vi "startup.vi"(8 "error in (no error)":errorcluster, 11 "ActionEditor in":refnum<class "ActionEditor.lvclass">) -> (0 "error out":errorcluster, 3 "ActionEditor out":refnum<class "ActionEditor.lvclass">)   [LabVIEW 2011, in "Views.lvlib" / "ScriptEditor.lvlib" / "ActionEditor.lvclass"]
uses:
  ActionEditor.lvclass
  ActionEditor.lvclass/ActionEditor.ctl
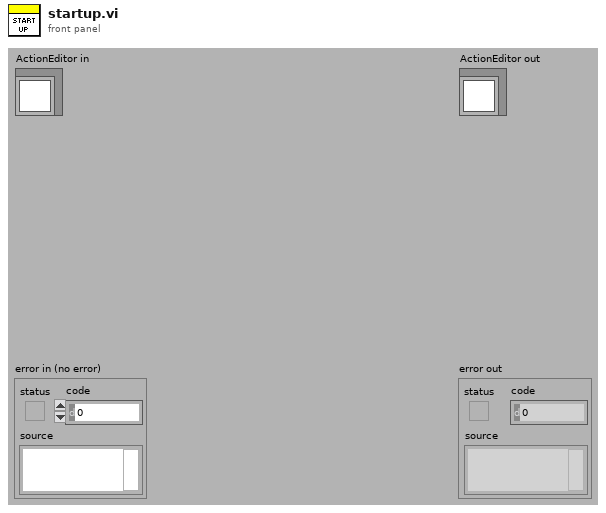
[diagram p1: front panel]
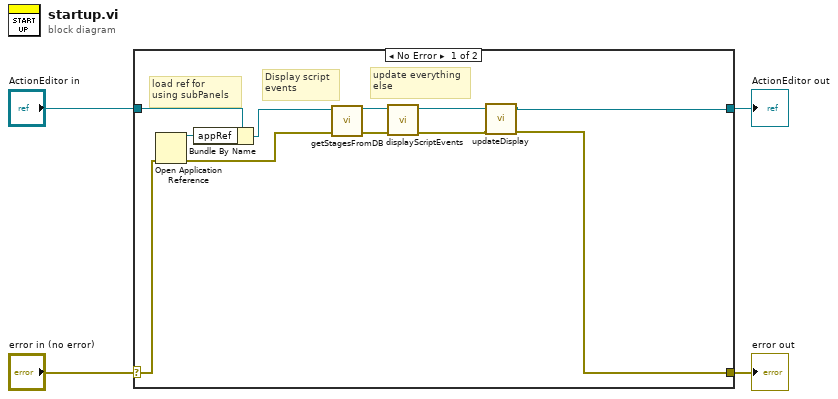
[diagram p0: block diagram]
diagram:
  n1 = case shown="No Error" "error in (no error)" {
    selector: "error in (no error)" -> [w12 w16]
    tunnel: [w7 w16] -> w3
    tunnel: [w8 w15] -> w1
    tunnel: "ActionEditor in" -> [w14 w15]
    frame No Error {
      # "update everything\nelse"
      # "Display script \nevents"
      # "load ref for\nusing subPanels"
      n2 = Open Application Reference(8:w12) -> (0:w11:errorcluster, 3:w13:refnum<vi>)  [unwired: 3 in]
      n3 = Bundle By Name(cluster=w14, "appRef"=w13) -> (w5:refnum<class "ActionEditor.lvclass">)
      n4 = call "getStagesFromDB.vi"("ActionEditor in"=w5) -> ("ActionEditor out"=w6:refnum<class "ActionEditor.lvclass">)  [unwired: 9 in, 1 out]
      n5 = call "displayScriptEvents.vi"("error in (no error)"=w11, "ActionEditor in"=w6) -> ("error out"=w9:errorcluster, "ActionEditor out"=w10:refnum<class "ActionEditor.lvclass">)  [unwired: 8 in]
      n6 = call "updateDisplay.vi"("error in (no error)"=w9, "ActionEditor in"=w10) -> ("error out"=w7:errorcluster, "ActionEditor out"=w8:refnum<class "ActionEditor.lvclass">)  [unwired: 8 in]
    }
    frame Error {
    }
  }
  "error out" <- w3
  "ActionEditor out" <- w1
